vi "Compressor_HW.vi"() -> ()   [LabVIEW 2017, in "Compressor.lvlib"]
uses:
  Compressor.lvlib
  Shared/TypeDef/Cluster_Compressor.ctl
  Globals/Global_STOP.vi
  Globals/GLOBAL_ACT Write_Data_Out.vi
panel:
  out "Compressor Running":bool
  out "Compressor Enabled":bool
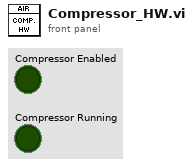
[diagram p1: front panel]
types:
  T1 = typedef "WPI_CompressorDevRef.ctl" = cluster{"DevStatus":errorcluster, "Pneumatics Control Module":u8}
  T2 = typedef "Cluster_Compressor.ctl" = cluster{"Compressor Running":bool, "Compressor Enabled":bool}
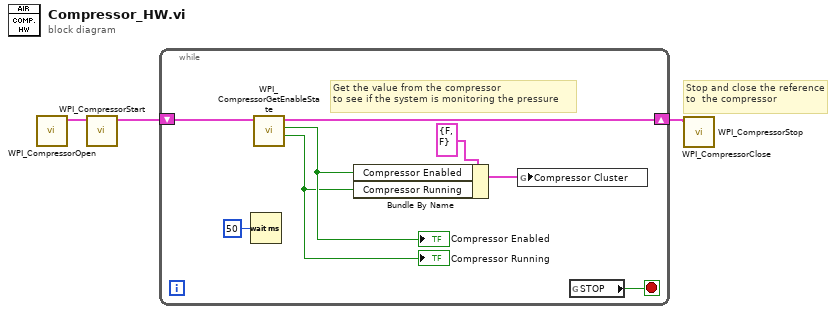
[diagram p0: block diagram]
diagram:
  # "Stop and close the reference to  the compressor"
  n1 = call <vilib>:"WPI_CompressorOpen.vi"() -> ("CompressorDevRef"=w2:T1)  [unwired: 14 in, 1 out]
  n2 = call <vilib>:"WPI_CompressorStart.vi"("CompressorDevRef"=w2) -> ("CompressorDevRef"=w3:T1)  [unwired: 1 in, 9 out]
  n3 = while {
    shift-right: [w11] -> w4
    shift-left: w3 -> [w12]
    stop <- w10 stop-if-true
    # "Get the value from the compressor \nto see if the system is monitoring the pressure"
    n4 = Wait (ms)(milliseconds to wait=u32 50) -> ()  [unwired: 1 out]
    n5 = call <vilib>:"WPI_CompressorGetEnableState.vi"("CompressorDevRef"=w12) -> ("Compressor Running"=w5:bool, "Enabled"=w6:bool, "CompressorDevRef"=w11:T1)  [unwired: 1 in, 7 out]
    "Compressor Enabled" <- w6
    "Compressor Running" <- w5
    n6 = Bundle By Name(cluster=T2 {"Compressor Running"=FALSE, "Compressor Enabled"=FALSE} ("Compressor Cluster"), "Compressor Enabled"=w6, "Compressor Running"=w5) -> (w7:T2)
    n7 = global write "GLOBAL_ACT Write_Data_Out.vi" "Compressor Cluster"(w7) -> ()
    n8 = global read "Global_STOP.vi" "STOP"() -> (w10:bool)
  }
  n9 = call <vilib>:"WPI_CompressorStop.vi"("CompressorDevRef"=w4) -> ("CompressorDevRef"=w1:T1)  [unwired: 1 in, 9 out]
  n10 = call <vilib>:"WPI_CompressorClose.vi"("CompressorDevRef"=w1) -> ()  [unwired: 1 in, 10 out]
